vi "Configure Comparator Beeper.vi"(8 "error in (no error)":errorcluster, 10 "Beeper Mode (0: Beep when Failed)":u16(ring) items=["Beep when Failed", "Beep when Pass"], 11 "VISA resource name":refnum<visa-resource-name>) -> (0 "error out":errorcluster, 3 "VISA resource name out":refnum<visa-resource-name>)   [LabVIEW 2016, in "Agilent E4980.lvlib"]
doc: "Selects the condition for generating a beeper sound: when sorting with the comparator fails (sorts into OUT OF BIN) or passes (sorts into BINs 1 to 9 or AUX BIN)."
uses:
  <instrlib>/Agilent E4980/Agilent E4980.lvlib
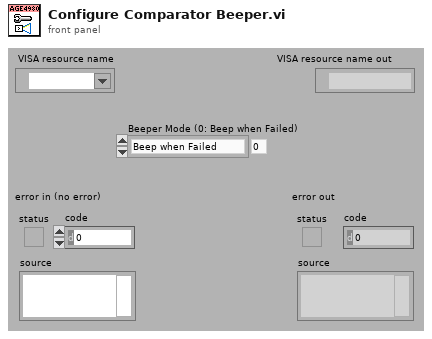
[diagram p1: front panel]
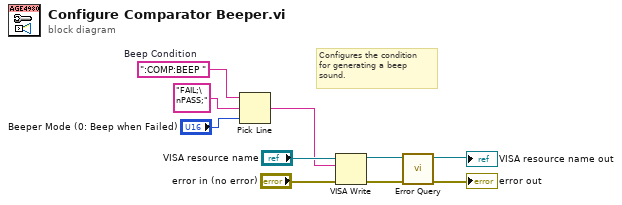
[diagram p0: block diagram]
diagram:
  w10 = ":COMP:BEEP "  # Beep Condition
  # "Configures the condition\nfor generating a beep\nsound."
  n1 = Pick Line(string ("")=w10, multi-line string="FAIL;\nPASS;", line index="Beeper Mode (0: Beep when Failed)") -> (output string=w5:string)
  n2 = VISA Write(VISA resource name="VISA resource name", write buffer=w5, error in (no error)="error in (no error)") -> (VISA resource name out=w4:refnum<visa-resource-name>, error out=w3:errorcluster)  [unwired: 1 out]
  n3 = call <instrlib>:"Error Query.vi"("error in (no error)"=w3, "VISA resource name"=w4) -> ("error out"=→"error out":errorcluster, "VISA resource name out"=→"VISA resource name out":refnum<visa-resource-name>)  [unwired: 6 in, 2 out]
